vi "extract_angles.vi"(0 "Ref point offset (mm)":dbl=100.1, 1 "XYZ in, two points":T1(array[cluster])) -> (3 "points out":T1(array[cluster]))   [LabVIEW 2010]
uses:
  utilities/labview/norm_vec.vi
panel:
  in  "Yaw axis":bool=TRUE
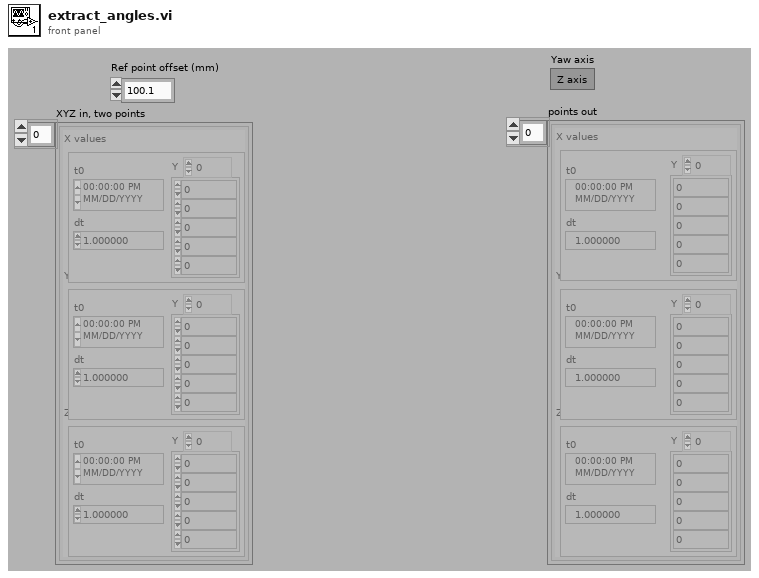
[diagram p1: front panel]
types:
  T1 = cluster{"X values":waveform(dbl), "Y values":waveform(dbl), "Z values":waveform(dbl)}[]
  T2 = cluster{"X values":waveform(dbl), "Y values":waveform(dbl), "Z values":waveform(dbl)}
  T3 = cluster{waveform(dbl), waveform(dbl), waveform(dbl)}
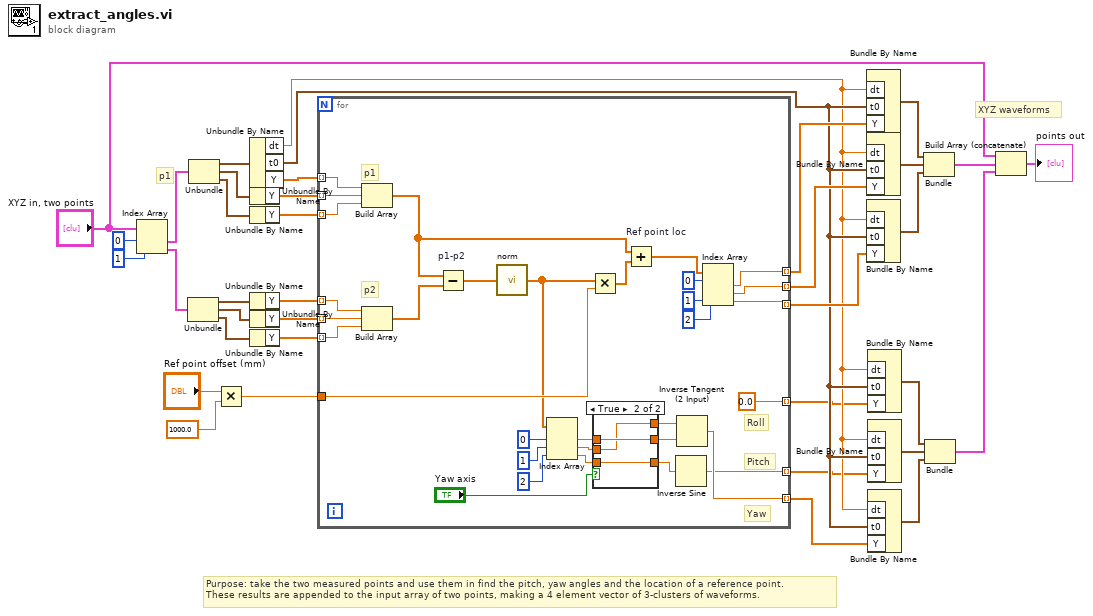
[diagram p0: block diagram]
diagram:
  # "Purpose: take the two measured points and use them in find the pitch, yaw angles and the location of a reference point.\nThese results are appended to the input array of two points, making a 4 element vector of 3-clusters of waveforms."
  # "XYZ waveforms"
  # "p1"
  n1 = Index Array(array="XYZ in, two points", index #1=0 ("index"), index #2=1 ("index")) -> (element #1=w35:T2, element #2=w26:T2)
  n2 = Unbundle(w26) -> ("X values"=w29:waveform(dbl), "Y values"=w28:waveform(dbl), "Z values"=w27:waveform(dbl))
  n3 = Unbundle(w35) -> ("X values"=w34:waveform(dbl), "Y values"=w33:waveform(dbl), "Z values"=w32:waveform(dbl))
  n4 = Multiply(x="Ref point offset (mm)", y=1000.0) -> (x*y=w2:dbl)
  n5 = Unbundle By Name(w34) -> ("dt"=w12:dbl, "t0"=w13:timestamp, "Y"=w22:dbl[])
  n6 = Unbundle By Name(w33) -> ("Y"=w30:dbl[])
  n7 = Unbundle By Name(w32) -> ("Y"=w31:dbl[])
  n8 = Unbundle By Name(w29) -> ("Y"=w25:dbl[])
  n9 = Unbundle By Name(w28) -> ("Y"=w24:dbl[])
  n10 = Unbundle By Name(w27) -> ("Y"=w23:dbl[])
  n11 = for {
    tunnel: w31 -> [w67] mode=indexing
    tunnel: w30 -> [w68] mode=indexing
    tunnel: w25 -> [w66] mode=indexing
    tunnel: w24 -> [w65] mode=indexing
    tunnel: w23 -> [w64] mode=indexing
    tunnel: w22 -> [w69] mode=indexing
    tunnel: [w59] -> w9 mode=indexing
    tunnel: [w58] -> w10 mode=indexing
    tunnel: w2 -> [w57]
    tunnel: [w53] -> w16 mode=indexing
    tunnel: [w52] -> w17 mode=indexing
    tunnel: [w51] -> w18 mode=indexing
    tunnel: [0.0] -> w11 mode=indexing
    # "Yaw"
    # "Pitch"
    # "Roll"
    # "p2"
    # "p1"
    n12 = Build Array(w69, w68, w67) -> (w41:dbl[])
    n13 = Build Array(w66, w65, w64) -> (w40:dbl[])
    n14 = Subtract "p1-p2"(x=w41, y=w40) -> (x-y=w39:dbl[])
    n15 = call-poly "norm.vi"("vector"=w39) -> ("normalized vector"=w38:dbl[])  [unwired: 4 out]
    n16 = Index Array(array=w38, index #1=0 ("index"), index #2=1 ("index"), index #3=2 ("index")) -> (element #1=w46:dbl, element #2=w44:dbl, element #3=w42:dbl)
    n17 = Multiply ("Multiply.vi")(x=w38, y=w57) -> (x*y=w63:dbl[])
    n18 = case shown="True" "Yaw axis" {
      tunnel: [w71 w75] -> w47
      tunnel: w46 -> [w72 w75]
      tunnel: [w70 w74] -> w45
      tunnel: w44 -> [w70 w74]
      tunnel: [w72 w73] -> w43
      tunnel: w42 -> [w71 w73]
      frame False {
      }
      frame True {
      }
    }
    n19 = Add "Ref point loc"(x=w41, y=w63) -> (x+y=w50:dbl[])
    n20 = Inverse Sine(1:w43) -> (0:w58:dbl)
    n21 = Inverse Tangent (2 Input)(1:w47, 2:w45) -> (0:w59:dbl)
    n22 = Index Array(array=w50, index #1=0 ("index"), index #2=1 ("index"), index #3=2 ("index")) -> (element #1=w53:dbl, element #2=w52:dbl, element #3=w51:dbl)
  }
  n23 = Bundle By Name("dt"=w12, "t0"=w13, "Y"=w16) -> (w21:waveform(dbl))  [unwired: 1 out]
  n24 = Bundle By Name("dt"=w12, "t0"=w13, "Y"=w17) -> (w20:waveform(dbl))  [unwired: 1 out]
  n25 = Bundle By Name("dt"=w12, "t0"=w13, "Y"=w18) -> (w19:waveform(dbl))  [unwired: 1 out]
  n26 = Bundle By Name("dt"=w12, "t0"=w13, "Y"=w11) -> (w8:waveform(dbl))  [unwired: 1 out]
  n27 = Bundle By Name("dt"=w12, "t0"=w13, "Y"=w10) -> (w7:waveform(dbl))  [unwired: 1 out]
  n28 = Bundle By Name("dt"=w12, "t0"=w13, "Y"=w9) -> (w6:waveform(dbl))  [unwired: 1 out]
  n29 = Bundle(w21, w20, w19) -> (w14:T3)  [unwired: 1 out]
  n30 = Bundle(w8, w7, w6) -> (w5:T3)  [unwired: 1 out]
  n31 = Build Array (concatenate)("XYZ in, two points", w14, w5) -> (→"points out":T1)
